vi "Add Test Case.vi"(8 "error in (no error)":errorcluster, 10 "Test Case":refnum<class "Test Case.lvclass">, 11 "Test Suite in":refnum<class "Test Suite.lvclass">) -> (0 "error out":errorcluster, 3 "Test Suite out":refnum<class "Test Suite.lvclass">)   [LabVIEW 2013, in "JUnit XML.lvlib" / "Test Suite.lvclass"]
doc: "Adds a test case to the test suite."
uses:
  Test Suite.lvclass
  Test Case/Test Case.lvclass
  Test Suite.lvclass/Test Suite.ctl
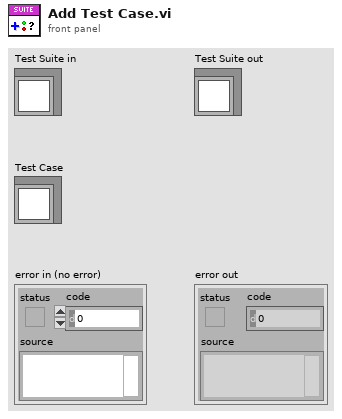
[diagram p1: front panel]
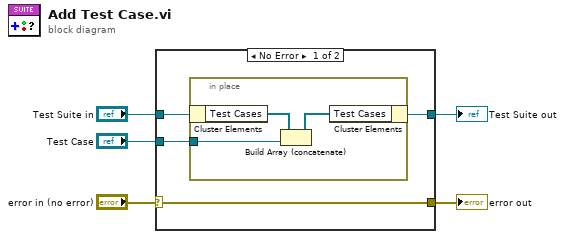
[diagram p0: block diagram]
diagram:
  n1 = case shown="No Error" "error in (no error)" {
    selector: "error in (no error)" -> [w9 w14]
    tunnel: [w9 w14] -> w4
    tunnel: [w7 w13] -> w2
    tunnel: "Test Suite in" -> [w8 w13]
    tunnel: "Test Case" -> [w6 _]
    frame No Error {
      n2 = in-place {
        in-place-border: w6 -> [w11]
        n3 = in-place-cluster #1(w8) -> ("Test Cases"=w12:refnum<class "Test Case.lvclass">[])
        n4 = Build Array (concatenate)(w12, w11) -> (w10:refnum<class "Test Case.lvclass">[])
        n5 = in-place-cluster #1("Test Cases"=w10) -> (w7:refnum<class "Test Suite.lvclass">)
      }
    }
    frame Error {
    }
  }
  "error out" <- w4
  "Test Suite out" <- w2
